vi "Deadzone.vi"(1 "Default":dbl, 2 "Deadzone":dbl, 3 "Input":dbl[](array[numeric])) -> (0 "Output":dbl[](array[numeric]))   [LabVIEW 2014]
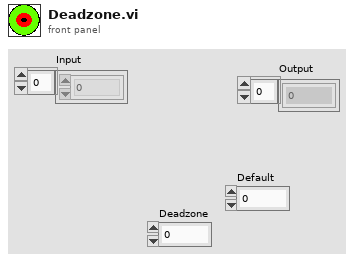
[diagram p1: front panel]
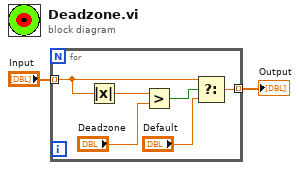
[diagram p0: block diagram]
diagram:
  n1 = for {
    tunnel: "Input" -> [w5] mode=indexing
    tunnel: [w3] -> w1 mode=indexing
    n2 = Absolute Value(x=w5) -> (abs(x)=w8:dbl)
    n3 = Greater?(x=w8, y="Deadzone") -> (0:w6:bool)
    n4 = Select(t=w5, s=w6, f="Default") -> (s? t:f=w3:dbl)
  }
  "Output" <- w1
